vi "FTW-Container-Update.vi"(0 "Object In":variant, 5 "Other Object":variant, 7 "Join Mode":T1, 11 "error in":errorcluster) -> (15 "error out":errorcluster)   [LabVIEW 2015]
uses:
  JSON/FTW-JSON-JoinMode.ctl
  <vilib>/Utility/Data Type/NI_Data Type.lvlib
panel:
  out "Updated Object":variant
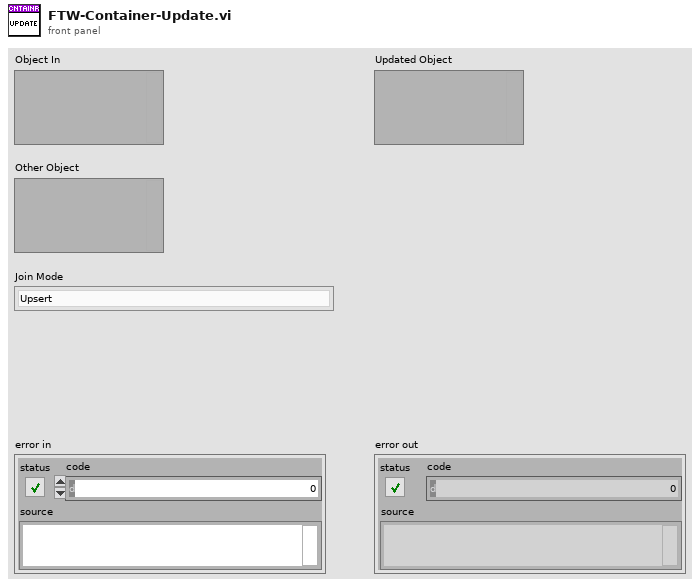
[diagram p1: front panel]
types:
  T1 = typedef "FTW-JSON-JoinMode.ctl" = enum32{"Upsert", "Update Only", "Insert Only"}
  T2 = typedef "NI_Data Type.lvlib/Data Type.ctl" = enum8{"Invalid Type", "Void", "I8", "I16", "I32", "I64", "U8", "U16", "U32", "U64", "Single Float", "Double Float", "Extended Float", "Single Complex", "Double Complex", "Extended Complex", "Enum U8", "Enum U16", "Enum U32", "Enum U64", "Single Float With Unit", "Double Float With Unit", "Extended Float With Unit", "Single Complex with Unit", "Double Complex with Unit", "Extended Complex with Unit", "Boolean", "String", "Path", "Picture", "Tag", "Array", "Cluster", "Variant", "LV Variant", "Waveform", "Timestamp", "Digital Waveform", "Digital Data", "ExpressData", "Refnum", "External Data", "VI", "Poly VI", "LabVIEW Class Instance", "Fixed Point"}
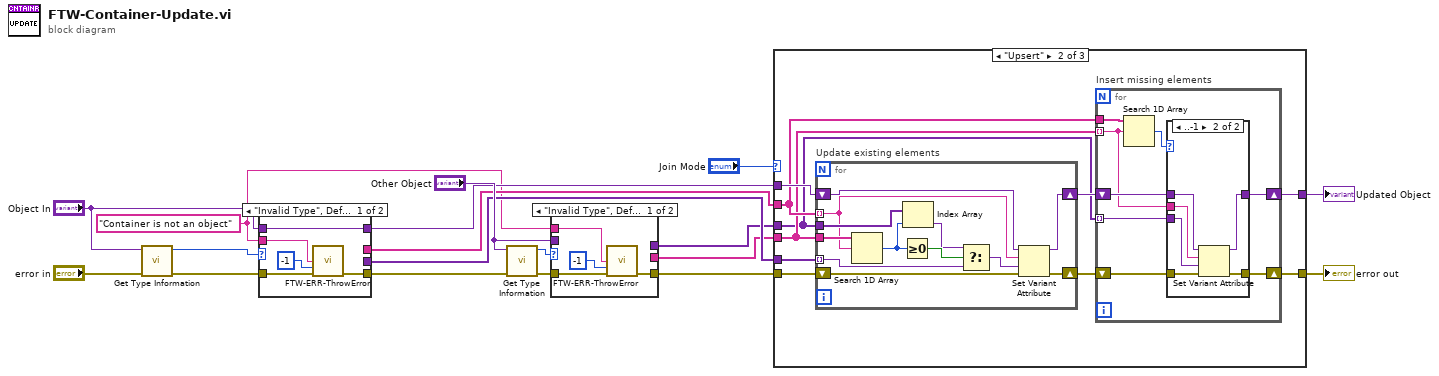
[diagram p0: block diagram]
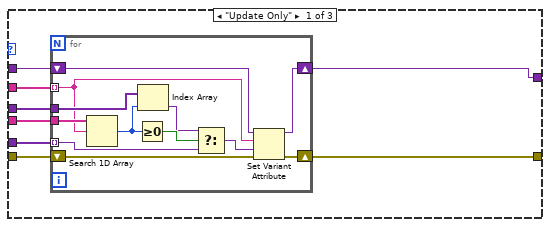
[diagram p2: hidden frame]
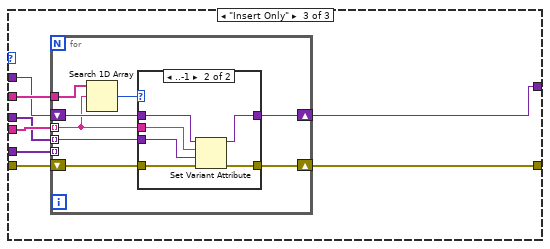
[diagram p4: hidden frame]
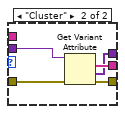
[diagram p6: hidden frame]
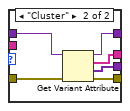
[diagram p7: hidden frame]
diagram:
  w1 = "Container is not an object" ("Error Message")
  n1 = call <vilib>:"Get Type Information.vi"("error in (no error)"="error in", "Variant"="Object In") -> ("error out"=w7:errorcluster, "Type"=w17:T2)  [unwired: 5 in, 3 out]
  n2 = case shown="\"Invalid Type\", Default" w17 {
    tunnel: "Object In" -> [w23 w29]
    tunnel: [_ w28] -> w13
    tunnel: [_ w27] -> w12
    tunnel: w7 -> [w22 w26]
    tunnel: [w23 w25] -> w6
    tunnel: [w21 w24] -> w3
    tunnel: w1 -> [w19 _]
    frame "Invalid Type", Default {
      n3 = call "FTW-ERR-ThrowError.vi"("Error Message"=w19, "Error Code"=-1, "error in"=w22) -> ("error out"=w21:errorcluster)  [unwired: 12 in]
    }
    frame "Cluster" {
      n4 = Get Variant Attribute(Variant=w29, error in=w26) -> (duplicate Variant=w25:variant, names=w28:string[], values=w27:variant[], error out=w24:errorcluster)  [unwired: 2 in]
    }
  }
  n5 = call <vilib>:"Get Type Information.vi"("error in (no error)"=w3, "Variant"="Other Object") -> ("error out"=w8:errorcluster, "Type"=w16:T2)  [unwired: 5 in, 3 out]
  n6 = case shown="\"Invalid Type\", Default" w16 {
    tunnel: "Other Object" -> [_ w38]
    tunnel: [_ w37] -> w11
    tunnel: [_ w36] -> w10
    tunnel: w8 -> [w33 w35]
    tunnel: [w32 w34] -> w2
    tunnel: w1 -> [w30 _]
    frame "Invalid Type", Default {
      n7 = call "FTW-ERR-ThrowError.vi"("Error Message"=w30, "Error Code"=-1, "error in"=w33) -> ("error out"=w32:errorcluster)  [unwired: 12 in]
    }
    frame "Cluster" {
      n8 = Get Variant Attribute(Variant=w38, error in=w35) -> (names=w37:string[], values=w36:variant[], error out=w34:errorcluster)  [unwired: 2 in, 1 out]
    }
  }
  n9 = case shown="\"Upsert\"" "Join Mode" {
    tunnel: w13 -> [w46 w61 w104]
    tunnel: w12 -> [w45 w68 w103]
    tunnel: w11 -> [w44 w60 w102]
    tunnel: w10 -> [w43 w59 w101]
    tunnel: w6 -> [w42 w67 w100]
    tunnel: [w41 w63 w99] -> w5
    tunnel: w2 -> [w40 w66 w98]
    tunnel: [w39 w62 w97] -> w4
    frame "Update Only" {
      n10 = for {
        tunnel: w46 -> [w51] mode=indexing
        tunnel: w45 -> [w53] mode=indexing
        tunnel: w44 -> [w58]
        tunnel: w43 -> [w57]
        shift-right: [w49] -> w41
        shift-left: w42 -> [w52]
        shift-right: [w47] -> w39
        shift-left: w40 -> [w48]
        n11 = Search 1D Array(1D array=w58, element=w51) -> (index of element=w56:i32)  [unwired: 1 in]
        n12 = Greater Or Equal To 0?(x=w56) -> (x >= 0?=w55:bool)
        n13 = Index Array(array=w57, index=w56) -> (element=w54:variant)
        n14 = Select(t=w54, s=w55, f=w53) -> (s? t:f=w50:variant)
        n15 = Set Variant Attribute(Variant=w52, name=w51, value=w50, error in=w48) -> (Variant out=w49:variant, error out=w47:errorcluster)  [unwired: 1 out]
      }
    }
    frame "Upsert" {
      n16 = for "Update existing elements" {
        tunnel: w61 -> [w89] mode=indexing
        tunnel: w68 -> [w91] mode=indexing
        tunnel: w60 -> [w96]
        tunnel: w59 -> [w95]
        shift-right: [w87] -> w65
        shift-left: w67 -> [w90]
        shift-right: [w85] -> w64
        shift-left: w66 -> [w86]
        n17 = Search 1D Array(1D array=w96, element=w89) -> (index of element=w94:i32)  [unwired: 1 in]
        n18 = Greater Or Equal To 0?(x=w94) -> (x >= 0?=w93:bool)
        n19 = Index Array(array=w95, index=w94) -> (element=w92:variant)
        n20 = Select(t=w92, s=w93, f=w91) -> (s? t:f=w88:variant)
        n21 = Set Variant Attribute(Variant=w90, name=w89, value=w88, error in=w86) -> (Variant out=w87:variant, error out=w85:errorcluster)  [unwired: 1 out]
      }
      n22 = for "Insert missing elements" {
        tunnel: w61 -> [w72]
        tunnel: w60 -> [w70] mode=indexing
        tunnel: w59 -> [w69] mode=indexing
        shift-right: [w75] -> w63
        shift-left: w65 -> [w76]
        shift-right: [w73] -> w62
        shift-left: w64 -> [w74]
        n23 = Search 1D Array(1D array=w72, element=w70) -> (index of element=w71:i32)  [unwired: 1 in]
        n24 = case shown="..-1" w71 {
          tunnel: w76 -> [w78 w84]
          tunnel: [w78 w83] -> w75
          tunnel: w74 -> [w77 w82]
          tunnel: [w77 w81] -> w73
          tunnel: w70 -> [_ w80]
          tunnel: w69 -> [_ w79]
          frame 0.. {
          }
          frame ..-1 {
            n25 = Set Variant Attribute(Variant=w84, name=w80, value=w79, error in=w82) -> (Variant out=w83:variant, error out=w81:errorcluster)  [unwired: 1 out]
          }
        }
      }
    }
    frame "Insert Only" {
      n26 = for {
        tunnel: w104 -> [w108]
        tunnel: w103 -> [_] mode=indexing
        tunnel: w102 -> [w106] mode=indexing
        tunnel: w101 -> [w105] mode=indexing
        shift-right: [w111] -> w99
        shift-left: w100 -> [w112]
        shift-right: [w109] -> w97
        shift-left: w98 -> [w110]
        n27 = Search 1D Array(1D array=w108, element=w106) -> (index of element=w107:i32)  [unwired: 1 in]
        n28 = case shown="..-1" w107 {
          tunnel: w112 -> [w114 w120]
          tunnel: [w114 w119] -> w111
          tunnel: w110 -> [w113 w118]
          tunnel: [w113 w117] -> w109
          tunnel: w106 -> [_ w116]
          tunnel: w105 -> [_ w115]
          frame 0.. {
          }
          frame ..-1 {
            n29 = Set Variant Attribute(Variant=w120, name=w116, value=w115, error in=w118) -> (Variant out=w119:variant, error out=w117:errorcluster)  [unwired: 1 out]
          }
        }
      }
    }
  }
  "error out" <- w4
  "Updated Object" <- w5
